vi "ADQ Control Unit Get Failed Device Count.vi"(8 "error in (no error)":errorcluster, 11 "adq_cu_ptr":u32) -> (0 "error out":errorcluster, 2 "function return":i32, 3 "adq_cu_ptr out":u32)   [LabVIEW 2013]
doc: "extern \"C\" __declspec(dllimport) int ADQControlUnit_GetFailedDeviceCount(void* adq_cu_ptr);"
uses:
  ADQAPI.dll
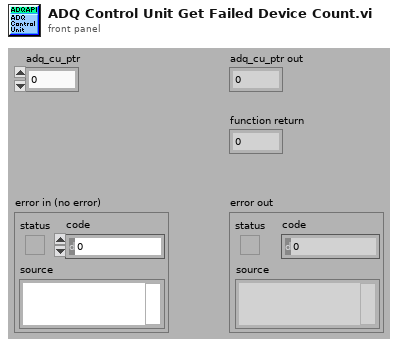
[diagram p1: front panel]
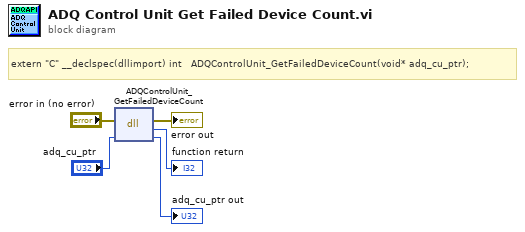
[diagram p0: block diagram]
diagram:
  # "extern \"C\" __declspec(dllimport) int\t\t\tADQControlUnit_GetFailedDeviceCount(void* adq_cu_ptr);"
  n1 = dll-call lib="C:/Users/astafiev/Desktop/Ilya/LabView_Radion/ADQAPI.*" fn="ADQControlUnit_GetFailedDeviceCount"(error in="error in (no error)", "adq_cu_ptr"="adq_cu_ptr") -> (error out=→"error out":errorcluster, "return type"=→"function return":i32, "adq_cu_ptr"=→"adq_cu_ptr out":u32)  [unwired: 2 in, 1 out]
